vi "Add_String.vi"(9 "Value":string, 10 "Key":string, 11 "Keyword Array":T1[](array[typedef])) -> (3 "Keyword Array Out":T1[](array[typedef]))   [LabVIEW 2013, in "Advanced Plotting Toolkit.lvlib"]
uses:
  Advanced Plotting Toolkit.lvlib
  KeyValue.ctl
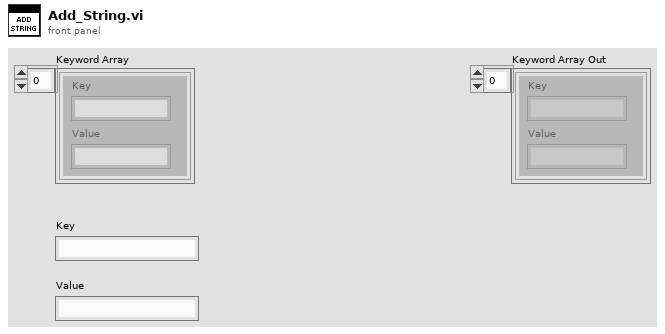
[diagram p1: front panel]
types:
  T1 = typedef "Advanced Plotting Toolkit.lvlib/KeyValue.ctl" = cluster{"Key":string, "Value":string}
  T2 = enum16{"big-endian, network order", "native, host order", "little-endian"}
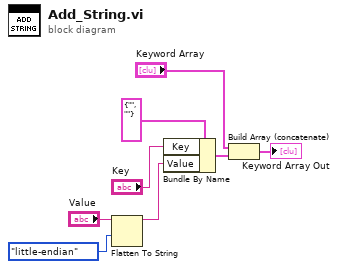
[diagram p0: block diagram]
diagram:
  n1 = Flatten To String(anything="Value", byte order (0:big-endian, network order)=T2."little-endian") -> (data string=w1:string)  [unwired: 2 in, 2 out]
  n2 = Bundle By Name(cluster=T1 {"Key"="", "Value"=""} ("KeyValue"), "Key"="Key", "Value"=w1) -> (w6:T1)
  n3 = Build Array (concatenate)("Keyword Array", w6) -> (→"Keyword Array Out":T1[])
